vi "Close all Client Connections.vi"(11 "Server Controller in":refnum<class "Server Controller.lvclass">) -> (3 "Server Controller out":refnum<class "Server Controller.lvclass">)   [LabVIEW 2013, in "Server Controller.lvlib" / "Server Controller.lvclass"]
uses:
  Server Controller.lvclass
  <vilib>/ActorFramework/Message Enqueuer/Message Enqueuer.lvclass
  Server Controller.lvclass/Server Controller.ctl
  <vilib>/ActorFramework/Message Enqueuer/Message Enqueuer.lvclass/Message Enqueuer.ctl
  <vilib>/ActorFramework/Message Enqueuer/Enqueue.vi
  <vilib>/ActorFramework/Message Priority Queue/Priority Enqueue.vi
  <vilib>/ActorFramework/Stop Msg/Stop Msg.lvclass
  <vilib>/NI/Actors/Linked Network Actor/Linked Network Actor Messages/Disconnect Msg/Disconnect Msg.lvclass
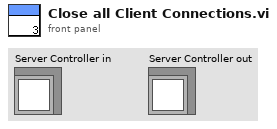
[diagram p1: front panel]
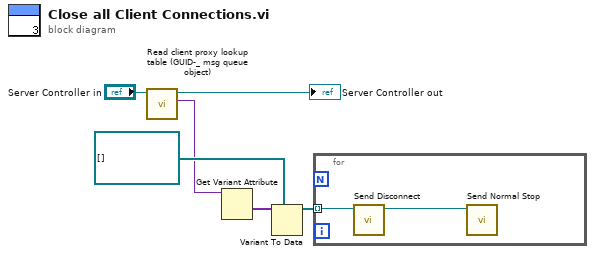
[diagram p0: block diagram]
diagram:
  n1 = call "Read client proxy lookup table (GUID-_ msg queue object).vi"("Server Controller in"="Server Controller in") -> ("client proxy lookup table (clientname -> msg queue object)"=w3:variant, "Server Controller out"=→"Server Controller out":refnum<class "Server Controller.lvclass">)  [unwired: 8 in, 1 out]
  n2 = Get Variant Attribute(Variant=w3) -> (values=w4:variant[])  [unwired: 3 in, 3 out]
  n3 = Variant To Data(type=refnum<class "Message Enqueuer.lvclass">[] [], Variant=w4) -> (data=w6:refnum<class "Message Enqueuer.lvclass">[])  [unwired: 1 in, 1 out]
  n4 = for {
    tunnel: w6 -> [w8] mode=indexing
    n5 = call <vilib>:"Send Disconnect.vi"("Message Enqueuer"=w8) -> ("Message Enqueuer out"=w7:refnum<class "Message Enqueuer.lvclass">)  [unwired: 9 in, 1 out]
    n6 = call <vilib>:"Send Normal Stop.vi"("Message Enqueuer"=w7) -> ()  [unwired: 10 in, 1 out]
  }
